vi "Configure VIs.Progress Window.Close.vi"(8 "error in (no error)":errorcluster, 10 "DVRs in":T1, 11 "VI refnum":refnum<vi>) -> (0 "error out":errorcluster)   [LabVIEW 2017]
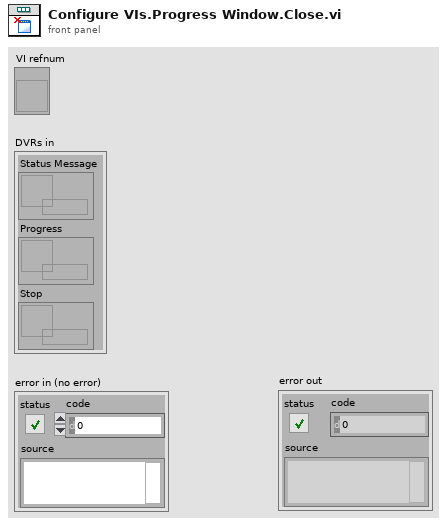
[diagram p1: front panel]
types:
  T1 = cluster{"Status Message":refnum<data-value>, "Progress":refnum<data-value>, "Stop":refnum<data-value>}
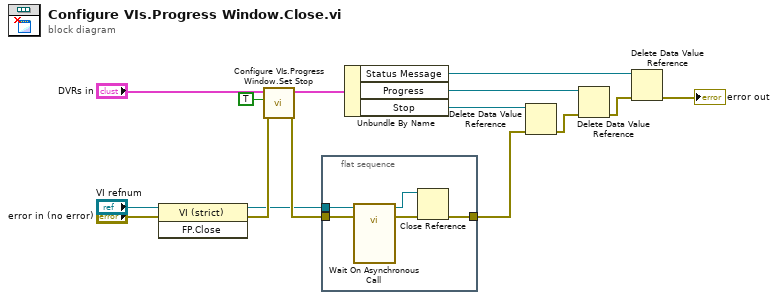
[diagram p0: block diagram]
diagram:
  n1 = invoke class="VI (strict)" method="FP.Close"(reference="VI refnum", error in="error in (no error)") -> (reference out=w1:refnum<vi>, error out=w2:errorcluster)  [unwired: 1 in, 1 out]
  n2 = call "Configure VIs.Progress Window.Set Stop.vi"("error in (no error)"=w2, "Stop"=TRUE, "DVRs in"="DVRs in") -> ("error out"=w5:errorcluster, "DVRs out"=w12:T1)  [unwired: 7 in]
  n3 = flat-sequence {
    tunnel: w1 -> [w17]
    tunnel: w5 -> [w16]
    tunnel: [w18] -> w7
    frame #0 {
      n4 = call-by-ref "Wait On Asynchronous Call"(reference=w17, error in=w16) -> (reference out=w20:refnum<vi>, error out=w19:errorcluster)  [unwired: 12 in]
      n5 = Close Reference(reference=w20, error in (no error)=w19) -> (error out=w18:errorcluster)
    }
  }
  n6 = Unbundle By Name(w12) -> ("Status Message"=w15:refnum<data-value>, "Progress"=w14:refnum<data-value>, "Stop"=w13:refnum<data-value>)
  n7 = Delete Data Value Reference(data value reference=w13, error in=w7) -> (error out=w8:errorcluster)  [unwired: 1 out]
  n8 = Delete Data Value Reference(data value reference=w14, error in=w8) -> (error out=w9:errorcluster)  [unwired: 1 out]
  n9 = Delete Data Value Reference(data value reference=w15, error in=w9) -> (error out=→"error out":errorcluster)  [unwired: 1 out]
